vi "inputView.vi"(10 "UserEvents in":refnum<class "UserEvents.lvclass">) -> ()   [LabVIEW 2013]
uses:
  UserEvents/UserEvents.lvclass
  Typedefs/ForceDemand.ctl
  <userlib>/Common/Devices/DistanceGauge/Typedefs/Distance Data.ctl
  Typedefs/ThermocoupleData.ctl
  UserEvents/UserEvents.lvclass/UserEvents.ctl
  Typedefs/StateSelector.ctl
  Typedefs/M2AADTTypedefs.lvlib
  <userlib>/Common/Devices/DistanceGauge/DistanceGauge.lvlib
panel:
  out "Thermocouple Data":T1={"Motor Temperature"=274.15} {"Motor Temperature" min=274.15 max=573.15 format="%.1f"}
  out "Distance Data":T2={"Distance Measured 1"=1.0, "Distance Measured 2"=1.0} {"Distance Measured 2" min=1.0 max=300.0 format="%.1f"; "Distance Measured 1" min=1.0 max=300.0 format="%.1f"}
  out "Force Measured":T3 min=-888.0 max=888.0 format="%.2f"
  out "SSI Encoder":i32
  out "2":bool
  out "1":bool
  # "Limit Switches"
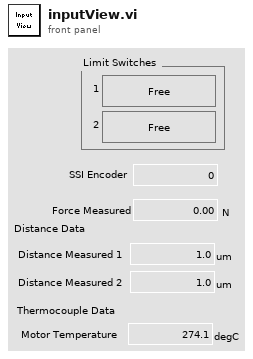
[diagram p1: front panel]
types:
  T1 = typedef "M2AADTTypedefs.lvlib/ThermocoupleData.ctl" = cluster{"Motor Temperature":dbl[unit]}
  T2 = typedef "DistanceGauge.lvlib/Distance Data.ctl" = cluster{"Distance Measured 1":dbl[unit], "Distance Measured 2":dbl[unit]}
  T3 = typedef "M2AADTTypedefs.lvlib/ForceDemand.ctl" = dbl[unit]
  T4 = typedef "M2AADTTypedefs.lvlib/PubDataEvents.ctl" = cluster{"State":refnum<user-event>, "ErrorCode":refnum<user-event>, "OutputData":refnum<user-event>, "InputData":refnum<user-event>, "ControllerData":refnum<user-event>, "TestStatus":refnum<user-event>, "LogPath":refnum<user-event>, "StiffnessData":refnum<user-event>}
  T5 = cluster{"Event Registration Refnum":refnum<event-registration>, "Event Registration Refnum":refnum<event-registration>}
  T6 = typedef "M2AADTTypedefs.lvlib/StateSelector.ctl" = enum16{"EndingCycleState", "FaultState", "InteractiveMotionState", "MovingToNewForceState", "OffState", "PausingState", "StandbyState", "StoppedState"}
  T7 = typedef "ILCCommon.lvlib/ILCTypedefs.lvlib/LimitSwitches.ctl" = cluster{"1":bool, "2":bool}
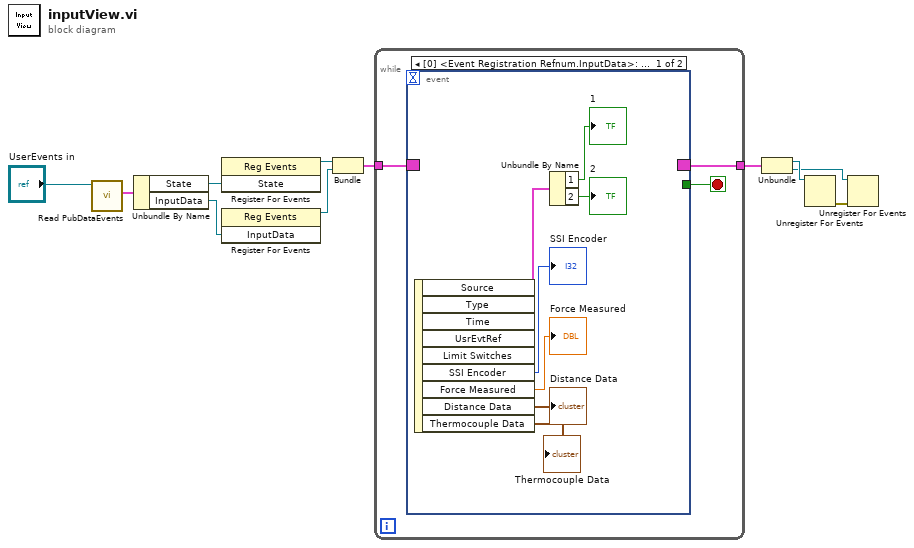
[diagram p0: block diagram]
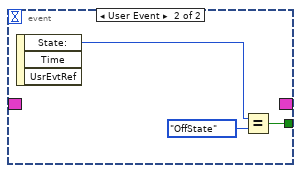
[diagram p2: hidden frame]
diagram:
  n1 = call "Read PubDataEvents.vi"("UserEvents in"="UserEvents in") -> ("PubDataEvents"=w11:T4)  [unwired: 9 in, 1 out]
  n2 = Unbundle By Name(w11) -> ("State"=w10:refnum<user-event>, "InputData"=w8:refnum<user-event>)
  n3 = register-events(w10) -> (reference out=w9:refnum<event-registration>)  [unwired: 2 in, 1 out]
  n4 = register-events(w8) -> (reference out=w7:refnum<event-registration>)  [unwired: 2 in, 1 out]
  n5 = Bundle("Event Registration Refnum"=w9, "Event Registration Refnum"=w7) -> (w5:T5)  [unwired: 1 in]
  n6 = while {
    tunnel: w5 -> [w14]
    tunnel: [w12] -> w4
    stop <- w13 stop-if-true
    n7 = event shown="[0] <Event Registration Refnum.InputData>: User Event" {
      selector: w14 -> [_ _]
      dyn-events: [_ _] -> w12
      timeout: _ -> [_ _]
      tunnel: [_ w23] -> w13
      event User Event {
        n8 = event-data() -> ("Limit Switches"=w21:T7, "SSI Encoder"=→"SSI Encoder":i32, "Force Measured"=→"Force Measured":T3, "Distance Data"=→"Distance Data":T2, "Thermocouple Data"=→"Thermocouple Data":T1)  [unwired: 1 in, 4 out]
        n9 = Unbundle By Name(w21) -> ("1"=→"1":bool, "2"=→"2":bool)
      }
      event User Event {
        n10 = event-data() -> ("State:"=w22:T6)  [unwired: 1 in, 2 out]
        n11 = Equal?(x=w22, y=StateSelector."OffState" ("State:")) -> (x = y?=w23:bool)
      }
    }
  }
  n12 = Unbundle(w4) -> ("Event Registration Refnum"=w3:refnum<event-registration>, "Event Registration Refnum"=w2:refnum<event-registration>)
  n13 = Unregister For Events(event registration refnum=w3) -> (error out=w1:errorcluster)  [unwired: 1 in]
  n14 = Unregister For Events(event registration refnum=w2, error in=w1) -> ()  [unwired: 1 out]
